vi "sub_qam_symbol_map_gen.vi"(9 "Gray code?":bool, 11 "M-QAM":i32) -> (3 "symbol map":cdb[](array[numeric]))   [LabVIEW 2014]
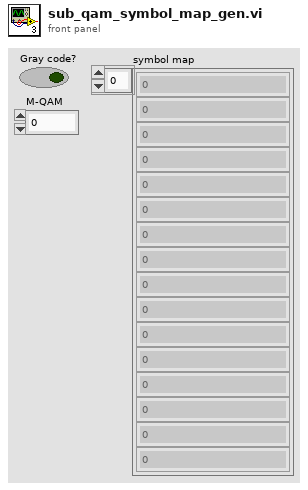
[diagram p1: front panel]
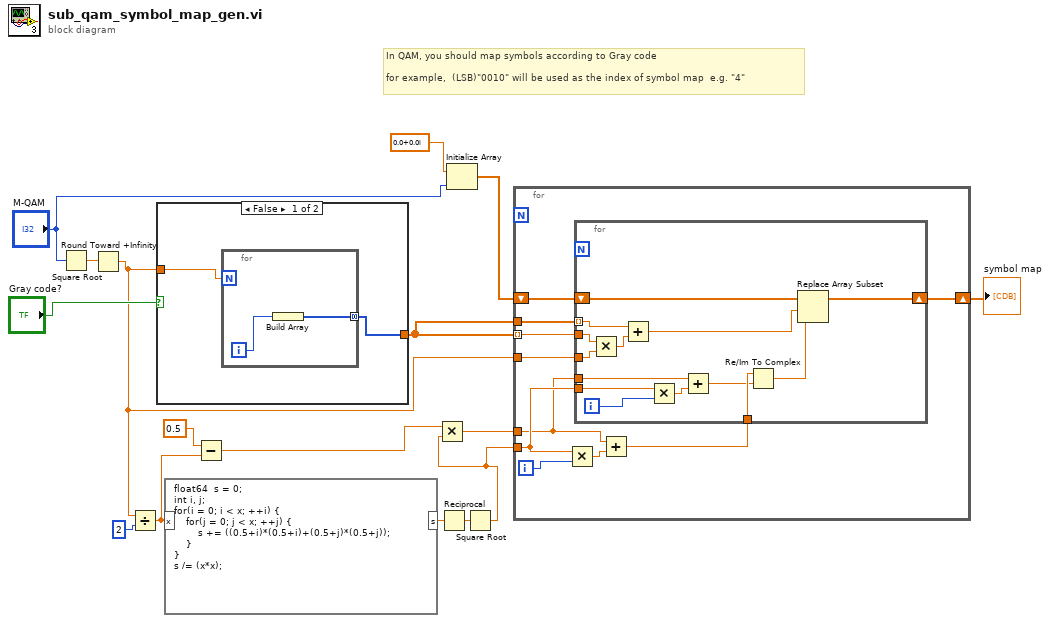
[diagram p0: block diagram]
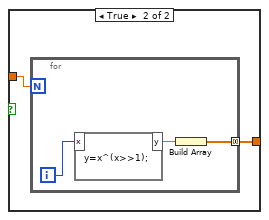
[diagram p2: hidden frame]
diagram:
  # "In QAM, you should map symbols according to Gray code\n\nfor example,  (LSB)\"0010\" will be used as the index of symbol map  e.g. \"4\""
  n1 = Square Root(x="M-QAM") -> (sqrt(x)=w11:dbl)
  n2 = Round Toward +Infinity(x=w11) -> (ceil(x): smallest int >= x=w9:dbl)
  n3 = Divide(x=w9, y=2) -> (x/y=w1:dbl)
  n4 = case shown="False" "Gray code?" {
    tunnel: w9 -> [w18 w22]
    tunnel: [w17 w21] -> w12
    frame False {
      n5 = for {
        N: w18 -> [_]
        tunnel: [w19] -> w17 mode=concatenating
        i -> [w20]
        n6 = Build Array(w20) -> (w19:i32[])
      }
    }
    frame True {
      n7 = for {
        N: w22 -> [_]
        tunnel: [w23] -> w21 mode=concatenating
        i -> [w25]
        n8 = formula code="y=x^(x>>1);"("x"=w25) -> ("y"=w24:dbl)
        n9 = Build Array(w24) -> (w23:dbl[])
      }
    }
  }
  n10 = formula code="float64  s = 0;\nint i, j;\nfor(i = 0; i < x; ++i) {\n    for(j = 0; j < x; ++j) {\n        s += ((0.5+i)*(0.5+i)+(0.5+j)*(0.5+j));\n    }\n}\ns /= (x*x);"("x"=w1) -> ("s"=w7:dbl)
  n11 = Subtract(x=0.5, y=w1) -> (x-y=w5:dbl)
  n12 = Reciprocal(x=w7) -> (1/x=w6:dbl)
  n13 = Initialize Array(cdb 0.0+0.0i, "M-QAM") -> (w14:cdb[])
  n14 = Square Root(x=w6) -> (sqrt(x)=w4:dbl)
  n15 = Multiply(x=w5, y=w4) -> (x*y=w3:dbl)
  n16 = for {
    tunnel: w12 -> [w33]
    shift-right: [w34] -> w10
    shift-left: w14 -> [w35]
    tunnel: w12 -> [w32] mode=indexing
    tunnel: w9 -> [w31]
    tunnel: w4 -> [w28]
    tunnel: w3 -> [w26]
    i -> [w30]
    n17 = Multiply(x=w28, y=w30) -> (x*y=w29:dbl)
    n18 = Add(x=w26, y=w29) -> (x+y=w27:dbl)
    n19 = for {
      shift-right: [w48] -> w34
      shift-left: w35 -> [w49]
      tunnel: w33 -> [w45] mode=indexing
      tunnel: w32 -> [w47]
      tunnel: w31 -> [w43]
      tunnel: w28 -> [w40]
      tunnel: w27 -> [w39]
      tunnel: w26 -> [w36]
      i -> [w41]
      n20 = Multiply(x=w47, y=w43) -> (x*y=w46:dbl)
      n21 = Add(x=w45, y=w46) -> (x+y=w44:dbl)
      n22 = Multiply(x=w40, y=w41) -> (x*y=w42:dbl)
      n23 = Add(x=w36, y=w42) -> (x+y=w38:dbl)
      n24 = Re/Im To Complex(1:w38, 2:w39) -> (0:w37:cdb)
      n25 = Replace Array Subset(array=w49, new element=w37, index=w44) -> (w48:cdb[])
    }
  }
  "symbol map" <- w10
